vi "zadanie_4.vi"() -> ()   [LabVIEW 2020]
panel:
  out "Cluster 2":T1
  in  "Cluster":T2
  # "Formularz"
  # "Dane"
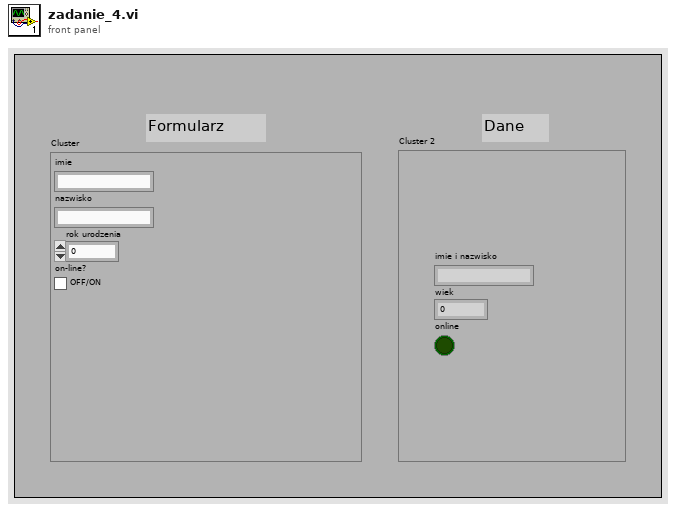
[diagram p1: front panel]
types:
  T1 = cluster{"imie i nazwisko":string, "wiek":dbl, "online":bool}
  T2 = cluster{"imie":string, "nazwisko":string, "rok urodzenia":dbl, "on-line?":bool}
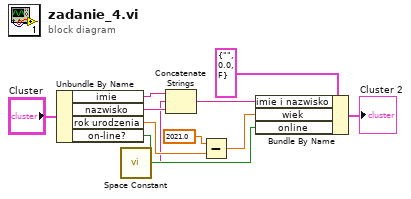
[diagram p0: block diagram]
diagram:
  n1 = Unbundle By Name("Cluster") -> ("imie"=w10:string, "nazwisko"=w2:string, "rok urodzenia"=w4:dbl, "on-line?"=w7:bool)
  n2 = call <vilib>:"Space Constant.vi"() -> ("String"=w1:string)
  n3 = Concatenate Strings(w10, w1, w2) -> (w9:string)
  n4 = Subtract(x=2021.0 ("y"), y=w4) -> (x-y=w8:dbl)
  n5 = Bundle By Name(cluster=T1 {"imie i nazwisko"="", "wiek"=0.0, "online"=FALSE} ("Cluster 2"), "imie i nazwisko"=w9, "wiek"=w8, "online"=w7) -> (→"Cluster 2":T1)
